vi "Config Type.vi"(11 "HighLimit Condition in":refnum<class "HighLimit Condition.lvclass">) -> (2 "Condition Config":refnum<class "Condition Config.lvclass">)   [LabVIEW 2020, in "VolatusSeq.lvlib" / "HighLimit Condition.lvclass"]
uses:
  HighLimit Condition.lvclass
  HighLimit Condition.lvclass/HighLimit Condition.ctl
  VolatusSeqConfig/HighLimit Condition Config/HighLimit Condition Config.lvclass
  C:/dev/lv20CE/relink/lv-volatus/VolatusSeqConfig/Condition Config/Condition Config.lvclass
  C:/dev/lv20CE/relink/lv-volatus/VolatusSeqConfig/HighLimit Condition Config/HighLimit Condition Config.lvclass
  VolatusSeqConfig/Condition Config/Condition Config.lvclass
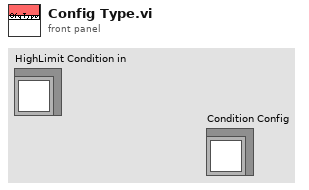
[diagram p1: front panel]
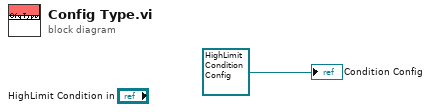
[diagram p0: block diagram]
diagram:
  "Condition Config" <- refnum<class "HighLimit Condition Config.lvclass"> refnum ("VolatusSeqConfig.lvlib:HighLimit Condition Config.lvclass")
